vi "Definitions FGV.vi"(8 "error in (no error)":errorcluster, 9 "Defintion Schema In":string, 10 "Definition Name":string, 11 "Action":T1) -> (0 "error out":errorcluster, 2 "Found?":bool, 3 "Definitions out":string)   [LabVIEW 2020, in "JSON Schema Generator.lvlib"]
uses:
  JSON Schema Generator.lvlib
  Defintion FGV Actions.ctl
  <vilib>/JDP Science/JSONtext/Next JSON Value.vi
  <vilib>/JDP Science/JSONtext/String Subset.vi
  <vilib>/JDP Science/JSONtext/Parsing/Advance past next JSON Value (inlined COPY).vi
  <vilib>/JDP Science/JSONtext/Parsing/Advance past whitespace.vi
  <vilib>/JDP Science/JSONtext/Parsing/Advance past String.vi
  <vilib>/JDP Science/JSONtext/Parsing/Advance past Number.vi
  <vilib>/JDP Science/JSONtext/Parsing/Advance past Line Ending.vi
  <vilib>/JDP Science/JSONtext/Parsing/Parse Full Path or Item Name.vi
  <vilib>/JDP Science/JSONtext/Parsing/Advance past Array.vi
  <vilib>/JDP Science/JSONtext/Parsing/Advance past Object.vi
  <vilib>/JDP Science/JSONtext/support/Error Cluster From Code.vi
  <vilib>/JDP Science/JSONtext/Offset/Find Item Locations by Path.vi
  <vilib>/JDP Science/JSONtext/JSONtext.lvlib
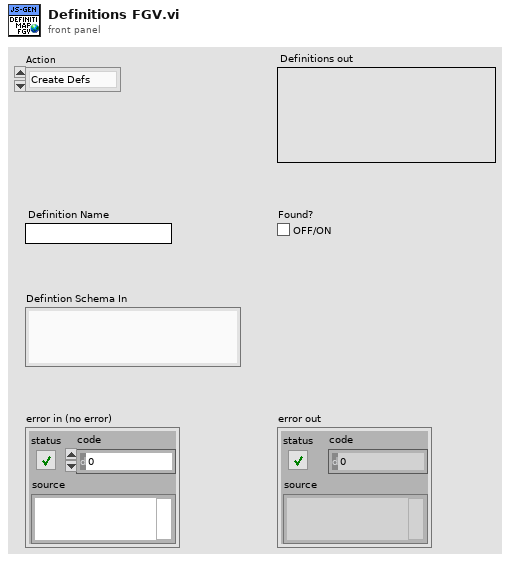
[diagram p1: front panel]
types:
  T1 = typedef "JSON Schema Generator.lvlib/Defintion FGV Actions.ctl" = enum16{"Create Defs", "Update Defs", "Get all Defs", "Get Def"}
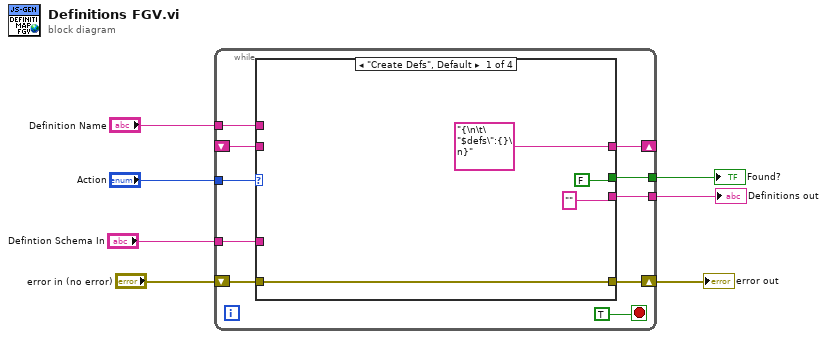
[diagram p0: block diagram]
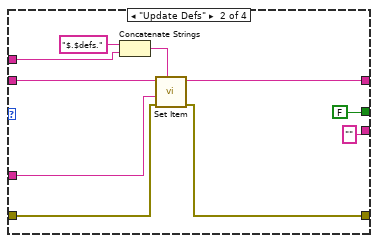
[diagram p2: hidden frame]
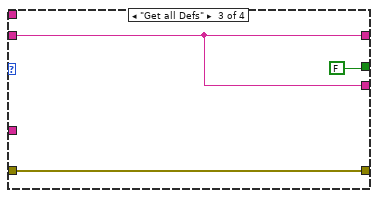
[diagram p3: hidden frame]
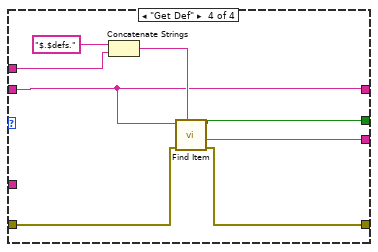
[diagram p4: hidden frame]
diagram:
  n1 = while {
    shift-right: [w15] -> _
    shift-left: _ -> [w14]
    tunnel: "Action" -> [w17]
    tunnel: [w13] -> w6
    tunnel: "Definition Name" -> [w12]
    shift-right: [w10] -> w3
    shift-left: "error in (no error)" -> [w11]
    tunnel: "Defintion Schema In" -> [w9]
    tunnel: [w8] -> w1
    stop <- TRUE stop-if-true
    n2 = case shown="\"Create Defs\", Default" w17 {
      tunnel: ["{\n\t\"$defs\":{}\n}" w30 w33 w39] -> w15
      tunnel: w14 -> [_ w29 w33 w39]
      tunnel: ["" ("<JSON>") "" w33 w38] -> w13
      tunnel: w12 -> [_ w26 _ w40]
      tunnel: w11 -> [w20 w25 w34 w36]
      tunnel: [w20 w24 w34 w37] -> w10
      tunnel: w9 -> [_ w23 _ _]
      tunnel: [FALSE ("Found") FALSE ("Found") FALSE ("Found") w35] -> w8
      frame "Create Defs", Default {
      }
      frame "Update Defs" {
        n3 = Concatenate Strings("$.$defs." ("$Path or Item Name"), w26) -> (w27:string)
        n4 = call <vilib>:"Set Item.vi"("$Path or Item Name"=w27, "error in (no error)"=w25, "JSON to Insert"=w23, "JSON"=w29) -> ("error out"=w24:errorcluster, "<JSON>"=w30:string)  [unwired: 4 in, 1 out]
      }
      frame "Get all Defs" {
      }
      frame "Get Def" {
        n5 = Concatenate Strings("$.$defs." ("$Path or Item Name"), w40) -> (w41:string)
        n6 = call <vilib>:"Find Item.vi"("$Path or Item Name"=w41, "error in (no error)"=w36, "JSON"=w39) -> ("error out"=w37:errorcluster, "<JSON>"=w38:string, "Found"=w35:bool)  [unwired: 5 in, 1 out]
      }
    }
  }
  "Definitions out" <- w6
  "error out" <- w3
  "Found?" <- w1
